vi "read nivstest file.vi"(8 "error in (no error)":errorcluster, 10 "lookup in":variant, 11 "Path":path=path "C:/Users/Public/Documents/National Instruments/NI VeriStand 2014/Projects/Example/Stimulus Profiles/Step Profile/Step Profile.nivstest") -> (0 "error out":errorcluster, 2 "lookup out":variant)   [LabVIEW 2014]
uses:
  <vilib>/Utility/sysdir.llb/System Directory Type.ctl
  <vilib>/xml/Load XML File.vi
  <vilib>/xml/Close Reference(Node).vi
  <vilib>/xml/NI_XML.lvlib
  <resource>/objmgr/DOMUserDefRef.rc
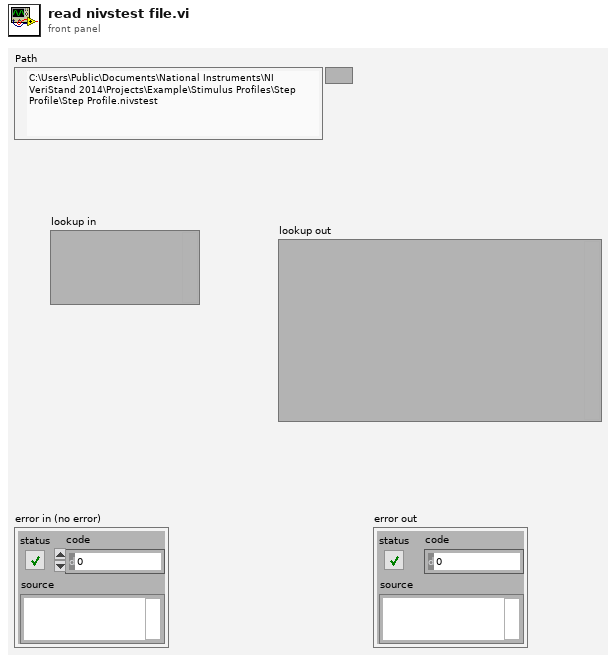
[diagram p1: front panel]
types:
  T1 = typedef "System Directory Type.ctl" = i32
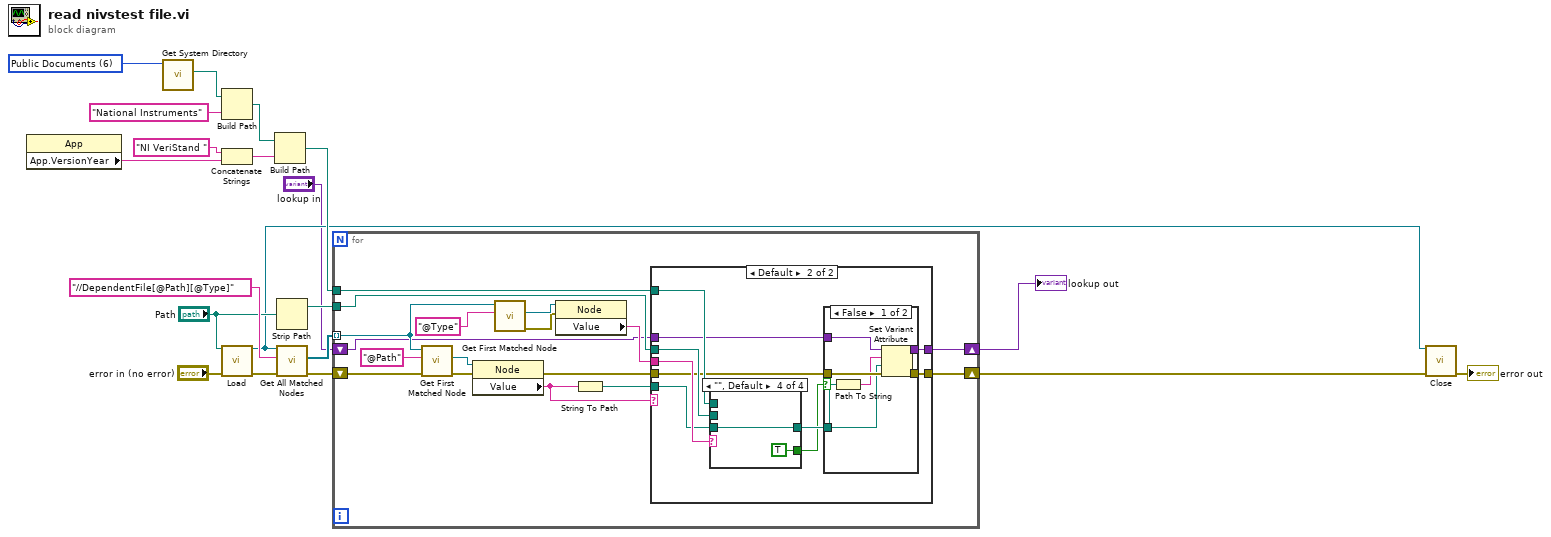
[diagram p0: block diagram]
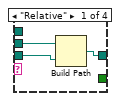
[diagram p4: hidden frame]
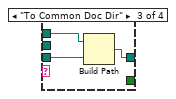
[diagram p6: hidden frame]
diagram:
  w12 = T1 6 items=["User Home"=0, "User Desktop"=1, "User Documents"=2, "User Application Data"=3, "User Preferences"=4, "User Temporary"=5, "Public Documents"=6, "Public Application Data"=7, "Public Preferences"=8, "Public Cache"=13, "System Core Libraries"=9, "System Installed Libraries"=10, "Application Files"=11, "Boot Volume Root"=12] ("system directory type")
  n1 = property class="App"() -> ("App.VersionYear"=w9:string)  [unwired: 2 in, 2 out]
  n2 = call <vilib>:"Get System Directory.vi"("system directory type"=w12) -> ("system directory"=w11:path)  [unwired: 10 in]
  n3 = Build Path(base path=w11, name or relative path="National Instruments") -> (appended path=w10:path)
  n4 = Concatenate Strings("NI VeriStand ", w9) -> (w6:string)
  n5 = call-poly <vilib>:"Load.vi"("path to XML document"="Path", "error in (no error)"="error in (no error)") -> ("DOM document out"=w3:refnum<k20>, "error out"=w18:errorcluster)  [unwired: 11 in, 1 out]
  n6 = Build Path(base path=w10, name or relative path=w6) -> (appended path=w5:path)
  n7 = Strip Path(path="Path") -> (stripped path=w13:path)  [unwired: 1 out]
  n8 = call <vilib>:"Get All Matched Nodes.vi"("error in (no error)"=w18, "XPath expression"="//DependentFile[@Path][@Type]", "node in"=w3) -> ("error out"=w15:errorcluster, "node result array"=w16:refnum<k20>[])  [unwired: 6 in, 1 out]
  n9 = for {
    tunnel: w16 -> [w29] mode=indexing
    shift-right: [w23] -> w4
    shift-left: w15 -> [w37]
    tunnel: w13 -> [w26]
    tunnel: w5 -> [w25]
    shift-right: [w21] -> w1
    shift-left: "lookup in" -> [w22]
    n10 = call <vilib>:"Get First Matched Node.vi"("error in (no error)"=w37, "XPath expression"="@Path", "node in"=w29) -> ("error out"=w35:errorcluster, "node result"=w34:refnum<k20>)  [unwired: 6 in, 1 out]
    n11 = property class="Node"(reference=w34, error in=w35) -> (error out=w24:errorcluster, "Value"=w33:string)  [unwired: 1 out]
    n12 = call <vilib>:"Get First Matched Node.vi"("XPath expression"="@Type", "node in"=w29) -> ("error out"=w31:errorcluster, "node result"=w32:refnum<k20>)  [unwired: 7 in, 1 out]
    n13 = property class="Node"(reference=w32, error in=w31) -> ("Value"=w28:string)  [unwired: 2 out]
    n14 = String To Path(string=w33) -> (path=w27:path)
    n15 = case shown="Default" w33 {
      tunnel: w28 -> [_ w49]
      tunnel: w27 -> [_ w48]
      tunnel: w26 -> [_ w47]
      tunnel: w25 -> [_ w46]
      tunnel: w24 -> [w39 w44]
      tunnel: [w39 w45] -> w23
      tunnel: w22 -> [w38 w42]
      tunnel: [w38 w41] -> w21
      frame "" {
      }
      frame Default {
        n16 = case shown="\"\", Default" w49 {
          tunnel: [w59 w61 w62 w66] -> w43
          tunnel: w48 -> [w58 w61 w63 w66]
          tunnel: w47 -> [w60 _ _ _]
          tunnel: w46 -> [_ _ w64 _]
          tunnel: [_ _ _ TRUE] -> w40
          frame "Relative" {
            n17 = Build Path(base path=w60, name or relative path=w58) -> (appended path=w59:path)
          }
          frame "Absolute" {
          }
          frame "To Common Doc Dir" {
            n18 = Build Path(base path=w64, name or relative path=w63) -> (appended path=w62:path)
          }
          frame "", Default {
          }
        }
        n19 = case shown="False" w40 {
          tunnel: [w55 w56] -> w45
          tunnel: w44 -> [w54 w56]
          tunnel: w43 -> [w53 _]
          tunnel: w42 -> [w51 w57]
          tunnel: [w50 w57] -> w41
          frame False {
            n20 = Path To String(path=w53) -> (string=w52:string)
            n21 = Set Variant Attribute(Variant=w51, name=w52, value=w53, error in=w54) -> (Variant out=w50:variant, error out=w55:errorcluster)  [unwired: 1 out]
          }
          frame True {
          }
        }
      }
    }
  }
  "lookup out" <- w1
  n22 = call-poly <vilib>:"Close.vi"("error in (no error)"=w4, "node"=w3) -> ("error out"=→"error out":errorcluster)  [unwired: 7 in]
